vi "ex4-9.vi"() -> ()   [LabVIEW 2009]
uses:
  <vilib>/NXT/Dual Mode Library/Display/drawNumber.vi
panel:
  in  "String":string
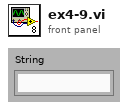
[diagram p1: front panel]
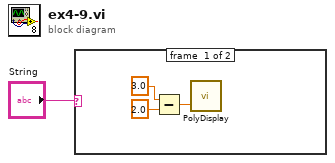
[diagram p0: block diagram]
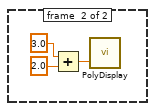
[diagram p2: hidden frame]
diagram:
  n1 = case shown="\" Add\"" "String" {
    frame #0 {
      n2 = Subtract(x=3.0, y=2.0) -> (x-y=w2:dbl)
      n3 = call-poly <vilib>:"PolyDisplay.vi"("number"=w2) -> ()  [unwired: 3 in, 1 out]
    }
    frame #1 {
      n4 = Add(x=3.0, y=2.0) -> (x+y=w5:dbl)
      n5 = call-poly <vilib>:"PolyDisplay.vi"("number"=w5) -> ()  [unwired: 3 in, 1 out]
    }
  }
